vi "webcom2.vi"() -> ()   [LabVIEW 2014]
uses:
  <vilib>/vision/NI_Vision_Development_Module.lvlib
panel:
  out "Image 7":T1(plugin-control)
  out "Image 6":T1(plugin-control)
  out "Image 5":T1(plugin-control)
  out "後":u32[][](array[numeric]) format="%x"
  out "Image 2":T1(plugin-control)
  out "Array":u32[][](array[colorbox])
  out "«e":u32[][](array[numeric]) format="%x"
  out "Image":T1(plugin-control)
  in  "Stop (F)":bool
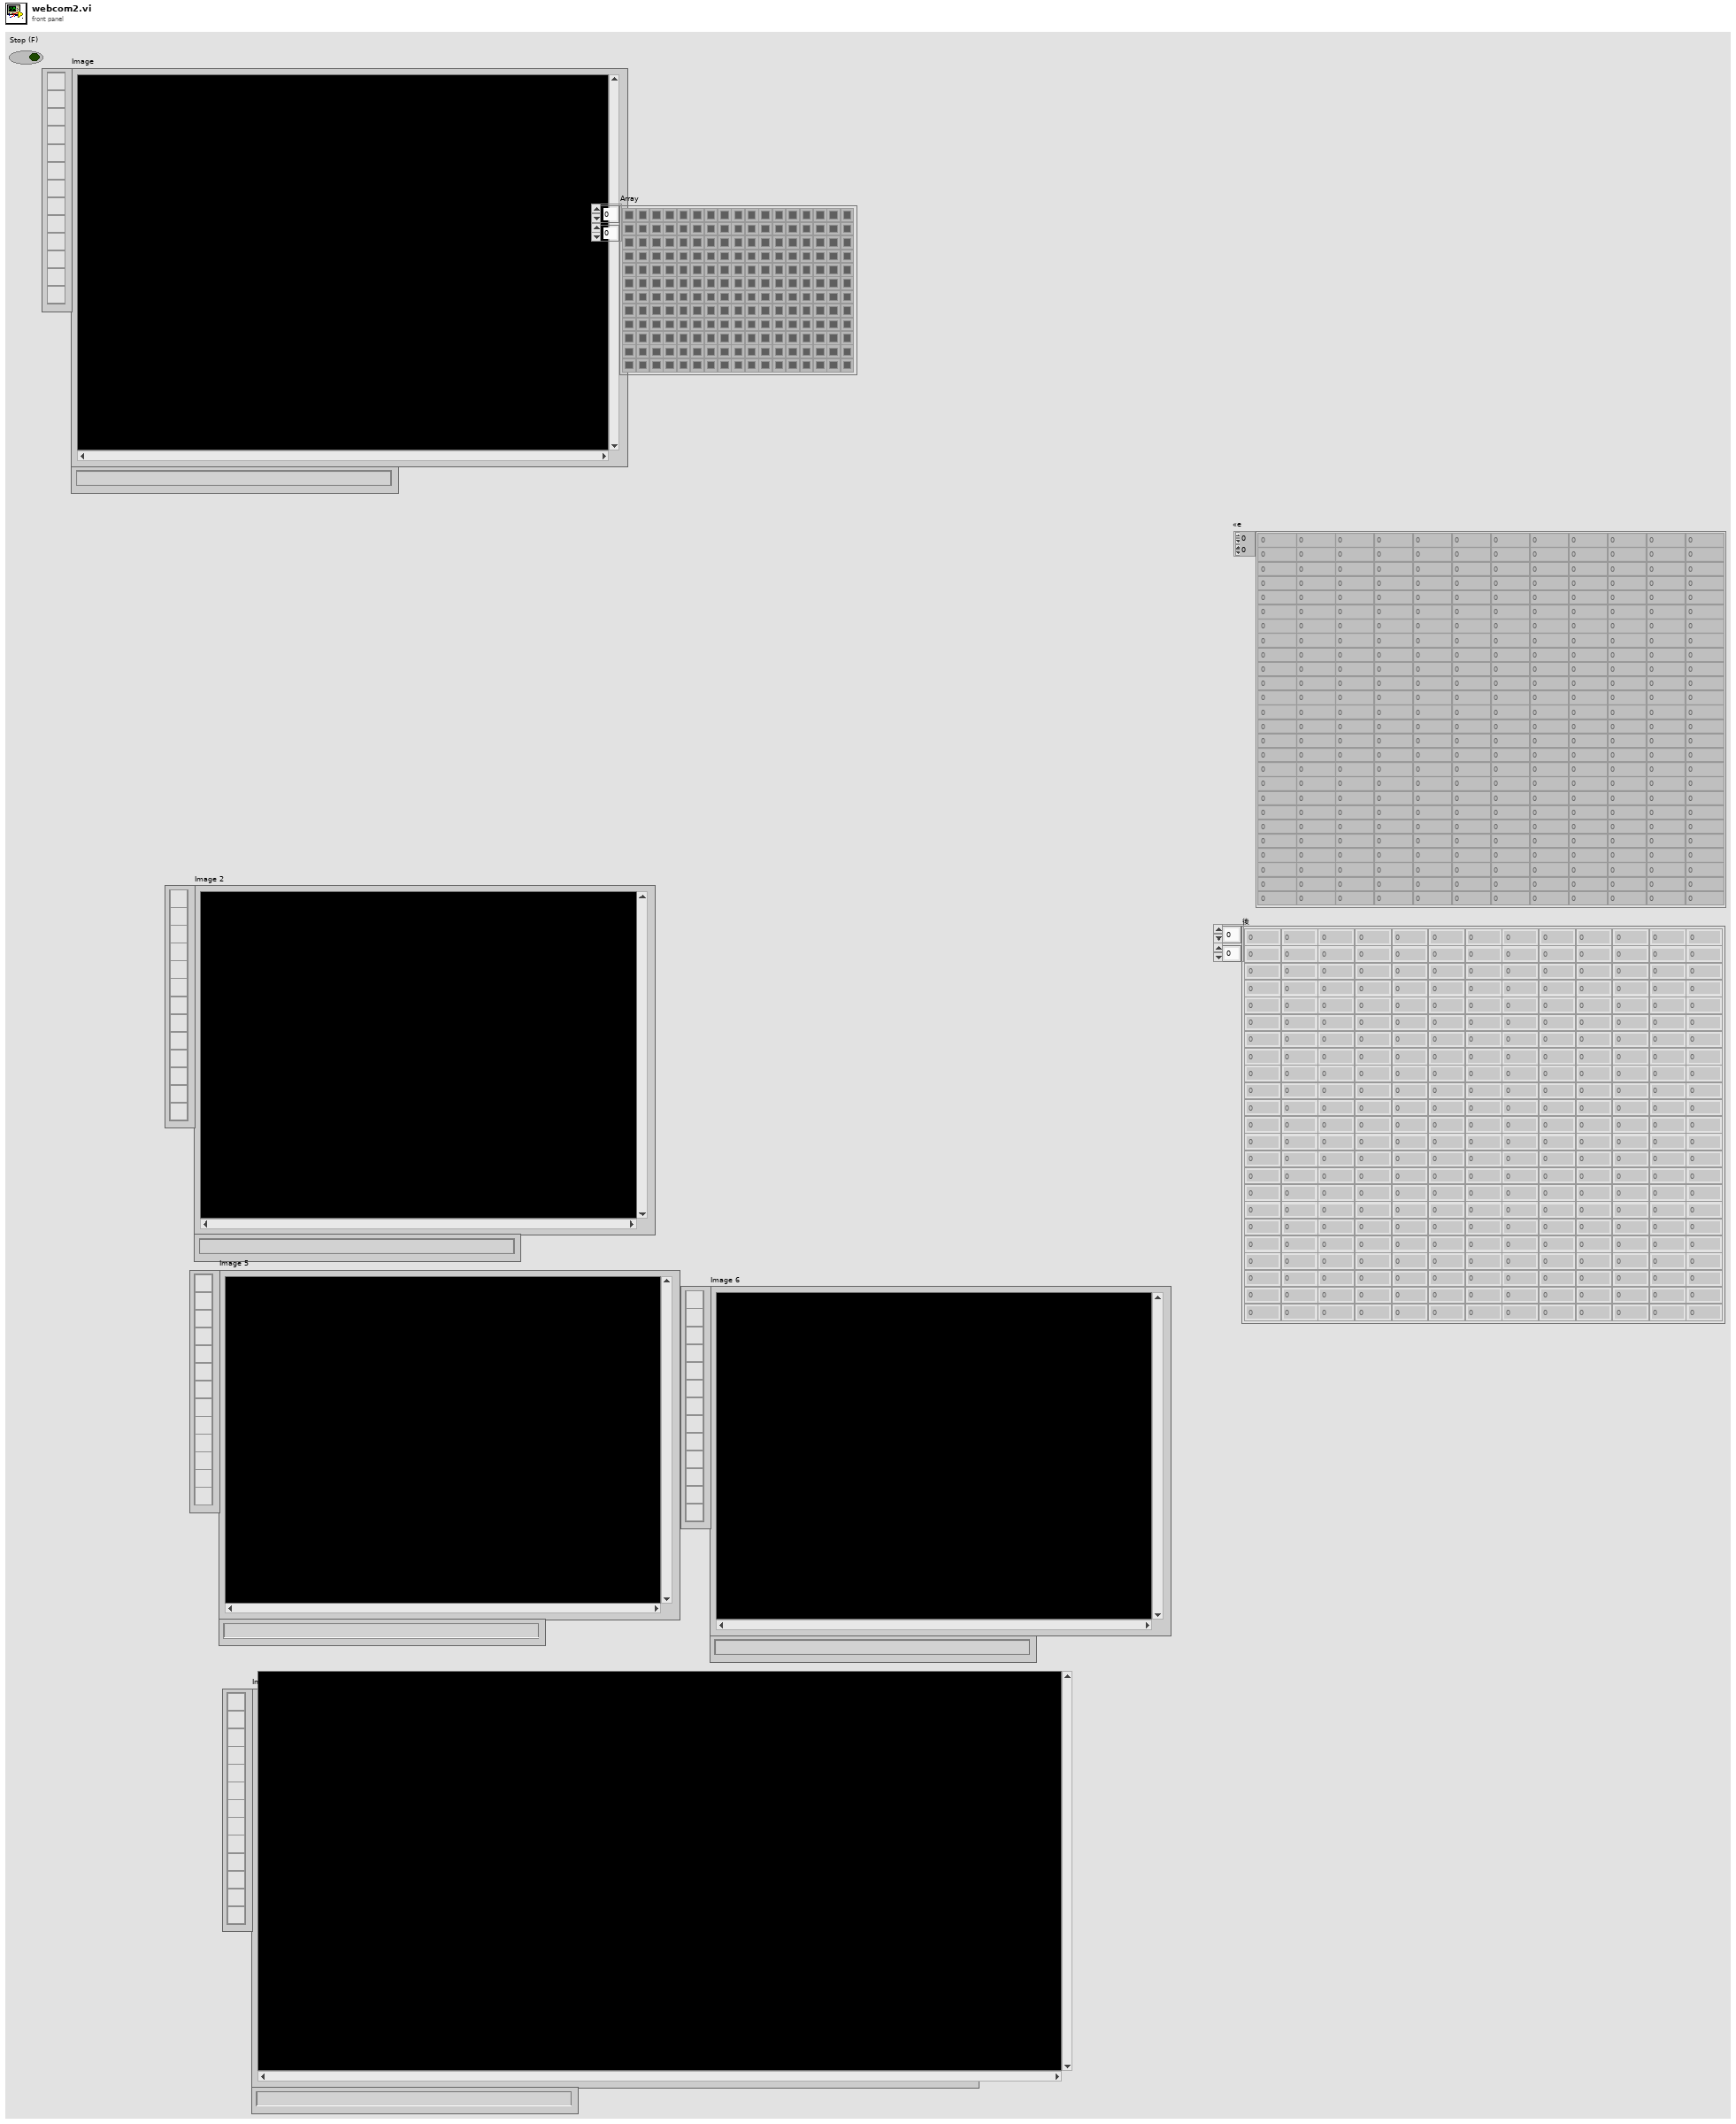
[diagram p1: front panel]
types:
  T1 = typedef "IMAQ Image.ctl" = refnum<image>
  T2 = typedef "Image Type" = u32
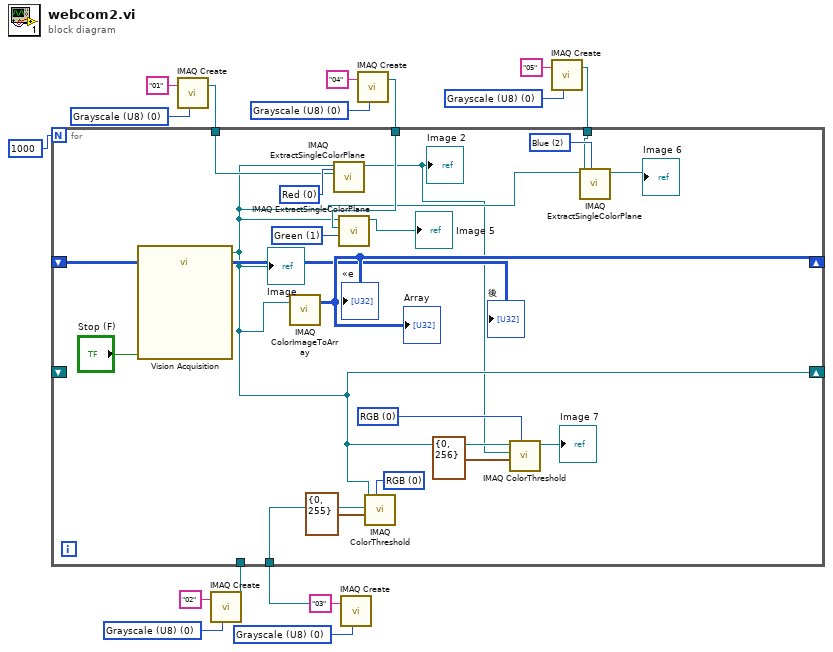
[diagram p0: block diagram]
diagram:
  w3 = T2 0 items=["Grayscale (U8)", "Grayscale (I16)", "Grayscale (SGL)", "Complex (CSG)", "RGB (U32)", "HSL (U32)", "RGB (U64)", "Grayscale (U16)"] ("Image Type")
  w5 = T2 0 items=["Grayscale (U8)", "Grayscale (I16)", "Grayscale (SGL)", "Complex (CSG)", "RGB (U32)", "HSL (U32)", "RGB (U64)", "Grayscale (U16)"] ("Image Type")
  w10 = T2 0 items=["Grayscale (U8)", "Grayscale (I16)", "Grayscale (SGL)", "Complex (CSG)", "RGB (U32)", "HSL (U32)", "RGB (U64)", "Grayscale (U16)"] ("Image Type")
  w12 = T2 0 items=["Grayscale (U8)", "Grayscale (I16)", "Grayscale (SGL)", "Complex (CSG)", "RGB (U32)", "HSL (U32)", "RGB (U64)", "Grayscale (U16)"] ("Image Type")
  w15 = T2 0 items=["Grayscale (U8)", "Grayscale (I16)", "Grayscale (SGL)", "Complex (CSG)", "RGB (U32)", "HSL (U32)", "RGB (U64)", "Grayscale (U16)"] ("Image Type")
  n1 = call "IMAQ Create"("Image Name"="01", "Image Type"=w15) -> ("New Image"=w16:T1)  [unwired: 3 in, 1 out]
  n2 = call "IMAQ Create"("Image Name"="02", "Image Type"=w12) -> ("New Image"=w11:T1)  [unwired: 3 in, 1 out]
  n3 = call "IMAQ Create"("Image Name"="03", "Image Type"=w10) -> ("New Image"=w8:T1)  [unwired: 3 in, 1 out]
  n4 = call "IMAQ Create"("Image Name"="04", "Image Type"=w5) -> ("New Image"=w4:T1)  [unwired: 3 in, 1 out]
  n5 = call "IMAQ Create"("Image Name"="05", "Image Type"=w3) -> ("New Image"=w1:T1)  [unwired: 3 in, 1 out]
  n6 = for {
    N: 1000 -> [_]
    tunnel: w16 -> [w30]
    shift-right: [w32] -> _
    shift-left: _ -> [w31]
    tunnel: w11 -> [_]
    tunnel: w8 -> [w27]
    shift-right: [w19] -> _
    shift-left: _ -> [_]
    tunnel: w4 -> [w24]
    tunnel: w1 -> [w20]
    w21 = 2 items=["Red", "Green", "Blue", "Hue", "Saturation", "Luminance", "Value", "Intensity"] ("Color Plane")
    w23 = 1 items=["Red", "Green", "Blue", "Hue", "Saturation", "Luminance", "Value", "Intensity"] ("Color Plane")
    w26 = u16 0 items=["RGB", "HSL", "HSV", "HSI"] ("Color Mode")
    w29 = u16 0 items=["RGB", "HSL", "HSV", "HSI"] ("Color Mode")
    w34 = 0 items=["Red", "Green", "Blue", "Hue", "Saturation", "Luminance", "Value", "Intensity"] ("Color Plane")
    n7 = call "Vision Acquisition"("Stop (F)"="Stop (F)") -> ("Image Out"=w19:T1)  [unwired: 24 in, 2 out]
    "Image" <- w19
    n8 = call "IMAQ ColorImageToArray"("Image"=w19) -> ("Image Pixels (U32)"=w32:u32[][])  [unwired: 3 in, 2 out]
    "«e" <- w32
    "Array" <- w32
    n9 = call "IMAQ ExtractSingleColorPlane"("Color Plane"=w34, "Image Dst"=w30, "Image Src"=w19) -> ("Image Dst Out"=w18:T1)  [unwired: 7 in, 1 out]
    "Image 2" <- w18
    n10 = call "IMAQ ExtractSingleColorPlane"("Color Plane"=w23, "Image Dst"=w24, "Image Src"=w19) -> ("Image Dst Out"=→"Image 5":T1)  [unwired: 7 in, 1 out]
    n11 = call "IMAQ ColorThreshold"("Color Mode"=w26, "Red or Hue Range"=cluster{"Lower value":i32, "Upper value":i32} {"Lower value"=0, "Upper value"=255}, "Image Dst"=w27, "Image Src"=w19) -> ()  [unwired: 6 in, 2 out]
    n12 = call "IMAQ ColorThreshold"("Color Mode"=w29, "Red or Hue Range"=cluster{"Lower value":i32, "Upper value":i32} {"Lower value"=0, "Upper value"=256}, "Image Dst"=w18, "Image Src"=w19) -> ("Image Dst Out"=→"Image 7":T1)  [unwired: 6 in, 1 out]
    n13 = call "IMAQ ExtractSingleColorPlane"("Color Plane"=w21, "Image Dst"=w20, "Image Src"=w19) -> ("Image Dst Out"=→"Image 6":T1)  [unwired: 7 in, 1 out]
    "後" <- w31
  }
